vi "AB_CheckApplicationDestinations.vi"(7 "Destination Path":path, 8 "error in (no error)":errorcluster, 10 "buildSpecName":string, 11 "buildObject":T1) -> (0 "error out":errorcluster, 2 "Checked base path":path)   [LabVIEW 2020]
uses:
  <resource>/Framework/Providers/API/ItemRef.ctl
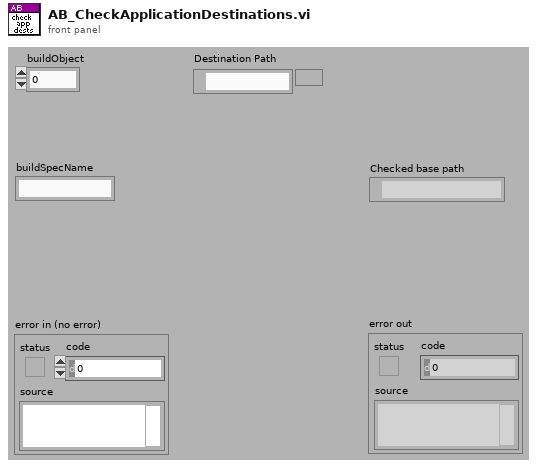
[diagram p1: front panel]
types:
  T1 = typedef "ItemRef.ctl" = u64
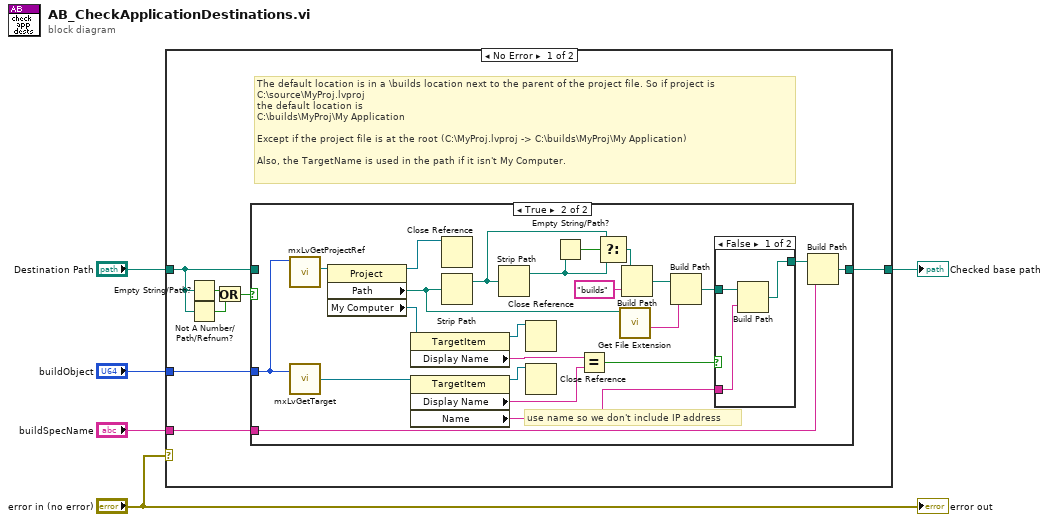
[diagram p0: block diagram]
diagram:
  n1 = case shown="No Error" "error in (no error)" {
    tunnel: "buildObject" -> [w12 _]
    tunnel: "buildSpecName" -> [w11 _]
    tunnel: [w10 _] -> w3
    tunnel: "Destination Path" -> [w7 _]
    frame No Error {
      # "The default location is in a \\builds location next to the parent of the project file. So if project is \nC:\\source\\MyProj.lvproj\nthe default location is \nC:\\builds\\MyProj\\My Application\n\nExcept if the project file is at the root (C:\\MyProj.lvproj -> C:\\builds\\MyProj\\My Application)\n\nAlso, the TargetName is used in the path if it isn't My Computer."
      n2 = Empty String/Path?(string/path=w7) -> (empty?=w9:bool)
      n3 = Not A Number/Path/Refnum?(number/path/refnum=w7) -> (NaN/Path/Refnum?=w8:bool)
      n4 = Or(x=w9, y=w8) -> (x .or. y?=w6:bool)
      n5 = case shown="True" w6 {
        tunnel: w12 -> [_ w25]
        tunnel: w11 -> [_ w29]
        tunnel: [w13 w26] -> w10
        tunnel: w7 -> [w13 _]
        frame False {
          # "The eventual API may allow building from a user defined path rather than relative to the project."
        }
        frame True {
          # "use name so we don't include IP address"
          n6 = call <resource>:"mxLvGetProjectRef.vi"("Item"=w25) -> ("Project Refnum"=w35:refnum<vi>)  [unwired: 1 in, 9 out]
          n7 = call <resource>:"mxLvGetTarget.vi"("Item"=w25) -> ("Target"=w21:refnum<vi>)  [unwired: 1 in, 2 out]
          n8 = property class="Project"(reference=w35) -> (reference out=w19:refnum<vi>, "Path"=w28:path, "My Computer"=w18:refnum<vi>)  [unwired: 1 in, 1 out]
          n9 = property class="TargetItem"(reference=w18) -> (reference out=w16:refnum<vi>, "Display Name"=w17:string)  [unwired: 1 in, 1 out]
          n10 = property class="TargetItem"(reference=w21) -> (reference out=w20:refnum<vi>, "Display Name"=w15:string, "Name"=w14:string)  [unwired: 1 in, 1 out]
          n11 = Close Reference(reference=w19) -> ()  [unwired: 1 in, 1 out]
          n12 = Strip Path(path=w28) -> (stripped path=w33:path)  [unwired: 1 out]
          n13 = Strip Path(path=w33) -> (stripped path=w32:path)  [unwired: 1 out]
          n14 = Close Reference(reference=w16) -> ()  [unwired: 1 in, 1 out]
          n15 = Close Reference(reference=w20) -> ()  [unwired: 1 in, 1 out]
          n16 = Empty String/Path?(string/path=w32) -> (empty?=w34:bool)
          n17 = Equal?(x=w17, y=w15) -> (x = y?=w22:bool)
          n18 = Select(t=w33, s=w34, f=w32) -> (s? t:f=w31:path)
          n19 = call <vilib>:"Get File Extension.vi"("file"=w28) -> ("filename without extension"=w27:string)  [unwired: 1 in, 9 out]
          n20 = Build Path(base path=w31, name or relative path="builds") -> (appended path=w30:path)
          n21 = Build Path(base path=w30, name or relative path=w27) -> (appended path=w24:path)
          n22 = case shown="False" w22 {
            tunnel: w24 -> [w39 w40]
            tunnel: [w38 w40] -> w23
            tunnel: w14 -> [w37 _]
            frame False {
              n23 = Build Path(base path=w39, name or relative path=w37) -> (appended path=w38:path)
            }
            frame True {
            }
          }
          n24 = Build Path(base path=w23, name or relative path=w29) -> (appended path=w26:path)
        }
      }
    }
    frame Error {
    }
  }
  "Checked base path" <- w3
  "error out" <- "error in (no error)"
